vi "RANGE File Setup.vi"(6 "Record":bool, 8 "Error In":errorcluster, 9 "Num Record":dbl, 10 "Create File":bool, 11 "Queue in":refnum<queue>) -> (0 "Error Out":errorcluster, 3 "Queue out":refnum<queue>)   [LabVIEW 2016]
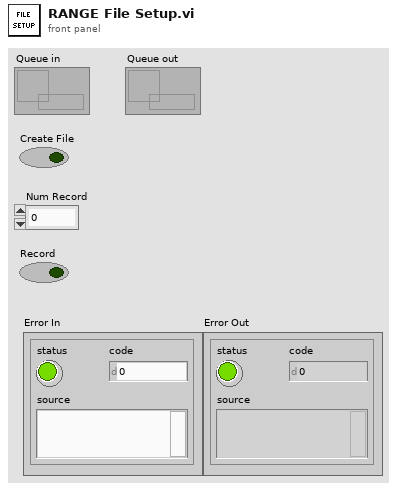
[diagram p1: front panel]
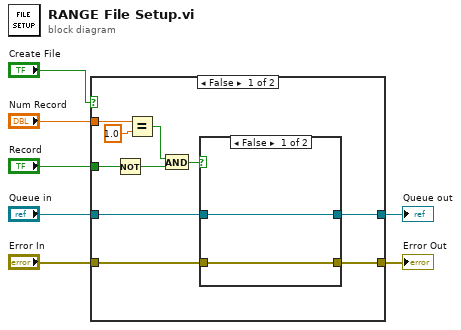
[diagram p0: block diagram]
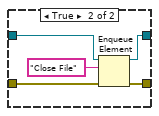
[diagram p2: hidden frame]
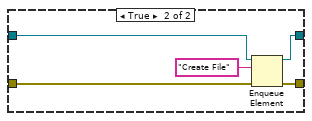
[diagram p3: hidden frame]
diagram:
  n1 = case shown="False" "Create File" {
    tunnel: "Queue in" -> [w16 w28]
    tunnel: [w15 w27] -> w4
    tunnel: "Record" -> [w11 _]
    tunnel: "Num Record" -> [w10 _]
    tunnel: [w8 w26] -> w2
    tunnel: "Error In" -> [w9 w25]
    frame False {
      n2 = Not(x=w11) -> (.not. x?=w12:bool)
      n3 = Equal?(x=w10, y=1.0) -> (x = y?=w14:bool)
      n4 = And(x=w14, y=w12) -> (x .and. y?=w13:bool)
      n5 = case shown="False" w13 {
        tunnel: w16 -> [w19 w23]
        tunnel: [w19 w22] -> w15
        tunnel: w9 -> [w18 w21]
        tunnel: [w18 w20] -> w8
        frame False {
        }
        frame True {
          n6 = Enqueue Element(queue=w23, element="Close File", error in (no error)=w21) -> (queue out=w22:refnum<queue>, error out=w20:errorcluster)  [unwired: 1 in, 1 out]
        }
      }
    }
    frame True {
      n7 = Enqueue Element(queue=w28, element="Create File", error in (no error)=w25) -> (queue out=w27:refnum<queue>, error out=w26:errorcluster)  [unwired: 1 in, 1 out]
    }
  }
  "Queue out" <- w4
  "Error Out" <- w2
